vi "CloseHardware.vi"(8 "error in (no error)":errorcluster, 11 "Point Grey Camera in":refnum<class "Point Grey Camera.lvclass">) -> (0 "error out":errorcluster, 3 "Point Grey Camera out":refnum<class "Point Grey Camera.lvclass">)   [LabVIEW 2020, in "Point Grey Camera.lvclass"]
uses:
  Point Grey Camera.lvclass
  Point Grey Camera.lvclass/Point Grey Camera.ctl
  NI_Vision_Acquisition_Software.lvlib
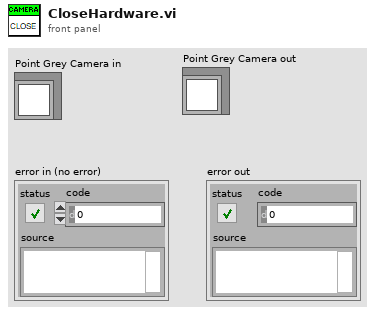
[diagram p1: front panel]
types:
  T1 = typedef "IMAQdx.ctl" = refnum<k21>
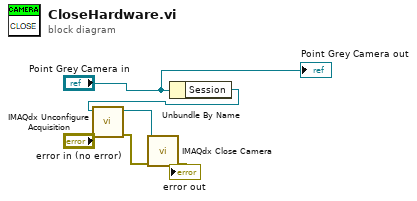
[diagram p0: block diagram]
diagram:
  n1 = Unbundle By Name("Point Grey Camera in") -> ("Session"=w6:T1)
  n2 = call "IMAQdx Unconfigure Acquisition.vi"("error in"="error in (no error)", "Session In"=w6) -> ("error out"=w4:errorcluster, "Session Out"=w3:T1)  [unwired: 8 in]
  n3 = call "IMAQdx Close Camera.vi"("error in"=w4, "Session In"=w3) -> ("error out"=→"error out":errorcluster)  [unwired: 9 in]
  "Point Grey Camera out" <- "Point Grey Camera in"
